vi "Ch1-Ex1.vi"() -> ()   [LabVIEW 2018]
panel:
  out "C":dbl
  in  "B":dbl
  in  "A":dbl
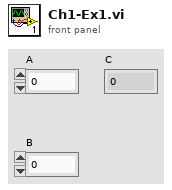
[diagram p1: front panel]
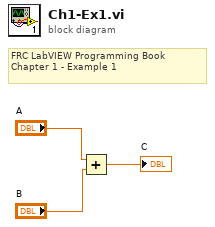
[diagram p0: block diagram]
diagram:
  # "FRC LabVIEW Programming Book\nChapter 1 - Example 1"
  n1 = Add(x="A", y="B") -> (x+y=→"C":dbl)
